vi "TotalVolumeFromDosageTimetable.vi"(11 "Zeitplan":string[][](table)) -> (2 "Volume T-2 [l]":dbl, 3 "Volume T-1 [l]":dbl)   [LabVIEW 2011]
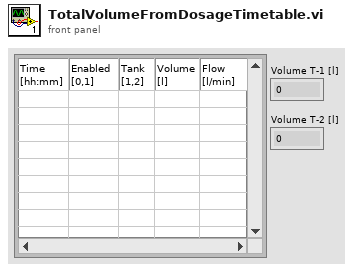
[diagram p1: front panel]
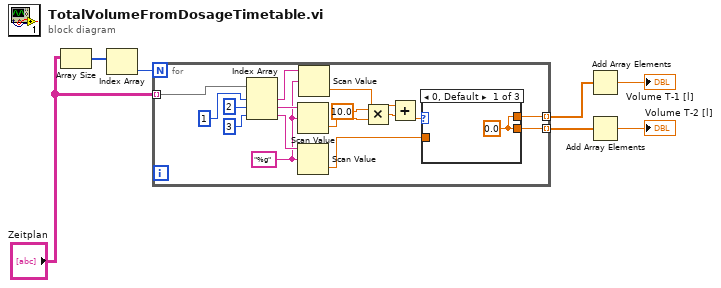
[diagram p0: block diagram]
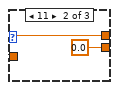
[diagram p2: hidden frame]
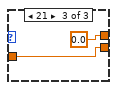
[diagram p3: hidden frame]
diagram:
  n1 = Array Size(array="Zeitplan") -> (size(s)=w5:i32[])
  n2 = Index Array(array=w5) -> (element=w4:i32)  [unwired: 1 in]
  n3 = for {
    N: w4 -> [_]
    tunnel: "Zeitplan" -> [w23] mode=indexing
    tunnel: [w18] -> w3 mode=indexing
    tunnel: [w16] -> w2 mode=indexing
    w13 = "%g" ("format string")
    n4 = Index Array(array=w23, index #1=1 ("index"), index #2=2 ("index"), index #3=3 ("index")) -> (element #1=w14:string, element #2=w19:string, element #3=w20:string)
    n5 = Scan Value(string=w19, format string=w13) -> (value=w12:dbl)  [unwired: 1 in, 1 out]
    n6 = Scan Value(string=w20, format string=w13) -> (value=w17:dbl)  [unwired: 1 in, 1 out]
    n7 = Scan Value(string=w14, format string=w13) -> (value=w8:dbl)  [unwired: 1 in, 1 out]
    n8 = Multiply(x=10.0, y=w12) -> (x*y=w10:dbl)
    n9 = Add(x=w8, y=w10) -> (x+y=w9:dbl)
    n10 = case shown="0, Default" w9 {
      tunnel: [w24 w26 0.0] -> w18
      tunnel: w17 -> [_ w26 w28]
      tunnel: [w24 0.0 w28] -> w16
      frame 0, Default {
        w24 = 0.0
      }
      frame 11 {
      }
      frame 21 {
      }
    }
  }
  n11 = Add Array Elements(numeric array=w3) -> (sum=→"Volume T-1 [l]":dbl)
  n12 = Add Array Elements(numeric array=w2) -> (sum=→"Volume T-2 [l]":dbl)
